vi "Determine Frame Timing Type.vi"(11 "GUID":string) -> (3 "CAN:Frame Type":T1)   [LabVIEW 2025, in "Protection and Counter Addon System Explorer.lvlib"]
uses:
  Protection and Counter Addon System Explorer.lvlib
  Types/CAN Filter Type.ctl
  Addon Shared/SubVIs/GUID Lookup.vi
  Addon Shared/Protection and Counter Addon Shared.lvlib
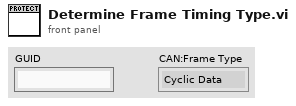
[diagram p1: front panel]
types:
  T1 = typedef "Protection and Counter Addon System Explorer.lvlib/CAN Filter Type.ctl" = enum16{"Cyclic Data", "Event Data", "Cyclic/Event", "All"}
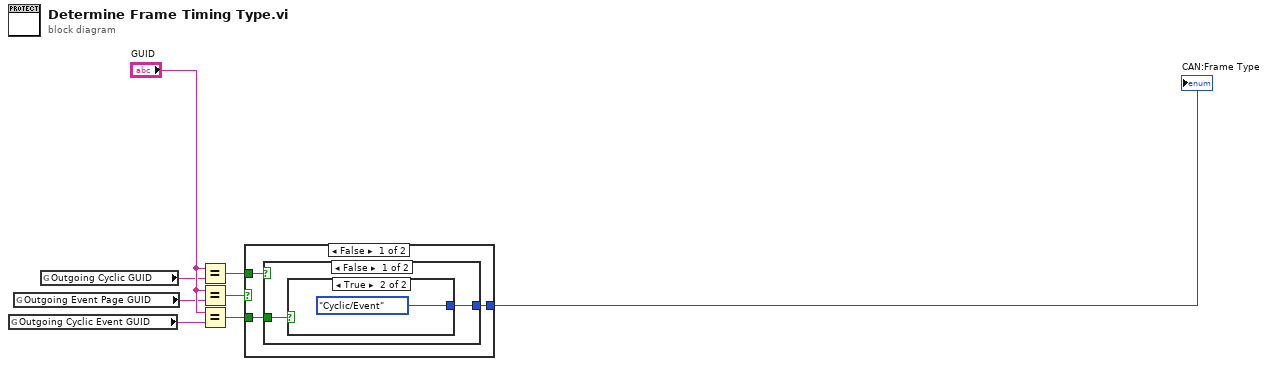
[diagram p0: block diagram]
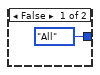
[diagram p2: hidden frame]
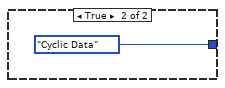
[diagram p3: hidden frame]
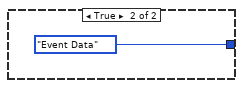
[diagram p4: hidden frame]
diagram:
  n1 = global read "GUID Lookup.vi" "Outgoing Cyclic Event GUID"() -> (w6:string)
  n2 = global read "GUID Lookup.vi" "Outgoing Event Page GUID"() -> (w5:string)
  n3 = global read "GUID Lookup.vi" "Outgoing Cyclic GUID"() -> (w4:string)
  n4 = Equal?(x="GUID", y=w4) -> (x = y?=w2:bool)
  n5 = Equal?(x="GUID", y=w5) -> (x = y?=w1:bool)
  n6 = Equal?(x="GUID", y=w6) -> (x = y?=w8:bool)
  n7 = case shown="False" w1 {
    tunnel: w2 -> [w11 _]
    tunnel: [w10 CAN_Filter_Type."Event Data" ("CAN:Frame Type")] -> w3
    tunnel: w8 -> [w9 _]
    frame False {
      n8 = case shown="False" w11 {
        tunnel: [w13 CAN_Filter_Type."Cyclic Data" ("CAN:Frame Type")] -> w10
        tunnel: w9 -> [w12 _]
        frame False {
          n9 = case shown="True" w12 {
            tunnel: [CAN_Filter_Type."All" ("CAN:Frame Type") CAN_Filter_Type."Cyclic/Event" ("CAN:Frame Type")] -> w13
            frame False {
            }
            frame True {
            }
          }
        }
        frame True {
        }
      }
    }
    frame True {
    }
  }
  "CAN:Frame Type" <- w3
